vi "RGBC_readColour.vi"(8 "error in (no error)":errorcluster, 10 "channel":enum16{"clear", "red", "green", "blue"}(ring), 11 "I2C Ref In":T1={"myRIO Reference"={"myRIO Model"=enum."Unknown", "myRIO Hardware Reference"={"Generic FPGA Reference"=refnum, "Allow multiple opens"=FALSE}}, "I2C Channels Enum"=enum."Not Connected", "I2C Configuration"={"I2C Transfer Rate"=enum."Fast mode (400 kbps)"}}) -> (0 "error out":errorcluster, 1 "value":u8, 2 "Bytes Read":u8[](array[numeric]), 3 "I2C Ref Out":T1={"myRIO Reference"={"myRIO Model"=enum."Unknown", "myRIO Hardware Reference"={"Generic FPGA Reference"=refnum, "Allow multiple opens"=FALSE}}, "I2C Channels Enum"=enum."Not Connected", "I2C Configuration"={"I2C Transfer Rate"=enum."Fast mode (400 kbps)"}})   [LabVIEW 2017]
uses:
  <vilib>/myRIO/Instrument Drivers/Onboard IO/I2C/typedefs/I2C Reference.ctl
  <vilib>/myRIO/Common/Instrument Driver Framework/Utilities/typedefs/myRIO Generic Hardware Reference.ctl
  <vilib>/myRIO/Common/Instrument Driver Framework/Utilities/typedefs/Hardware Version Enum.ctl
  <vilib>/myRIO/Common/Instrument Driver Framework/Utilities/typedefs/myRIO v1.0 Reference.ctl
  <vilib>/myRIO/Common/Instrument Driver Framework/Utilities/typedefs/Generic FPGA Reference.ctl
  <vilib>/myRIO/Common/Instrument Driver Framework/myRIO v1.0/I2C/typedefs/I2C Channels Enum.ctl
  <vilib>/myRIO/Instrument Drivers/Onboard IO/I2C/typedefs/I2C Configuration.ctl
  <vilib>/myRIO/Instrument Drivers/Onboard IO/I2C/typedefs/I2C Transfer Rate.ctl
  <vilib>/Utility/error.llb/Error Cluster From Error Code.vi
  <vilib>/myRIO/Common/Instrument Driver Framework/myRIO v1.0/I2C/vis/myRIO v1.0 Write I2C.vi
  <vilib>/myRIO/Common/Instrument Driver Framework/myRIO v1.0/I2C/vis/myRIO v1.0 Read I2C.vi
  <vilib>/myRIO/Instrument Drivers/Onboard IO/I2C/I2C.lvlib
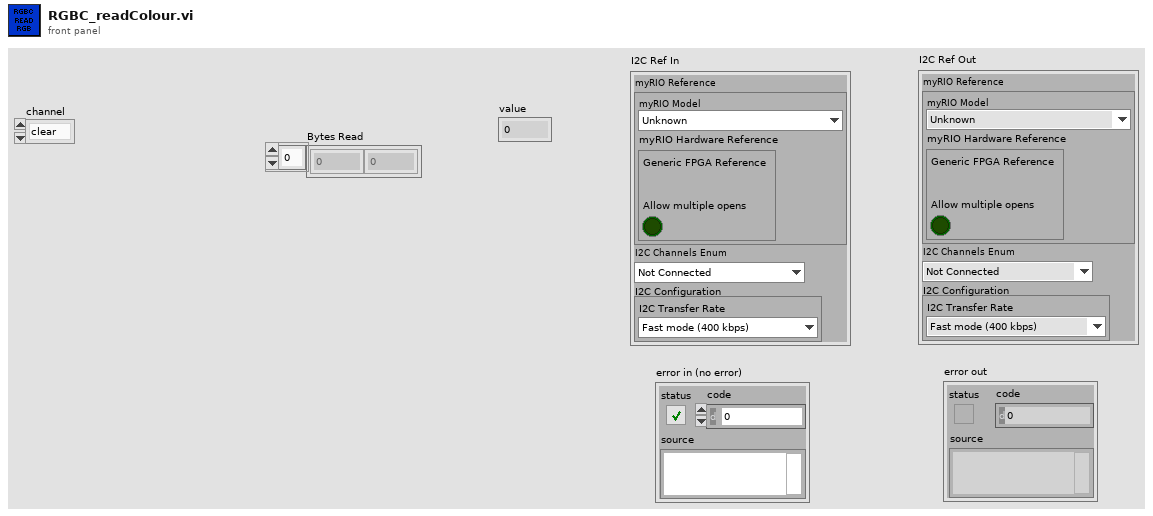
[diagram p1: front panel]
types:
  T1 = typedef "I2C.lvlib/I2C Reference.ctl" = cluster{"myRIO Reference":T2, "I2C Channels Enum":T6, "I2C Configuration":T7}
  T2 = typedef "myRIO Generic Hardware Reference.ctl" = cluster{"myRIO Model":T3, "myRIO Hardware Reference":T4}
  T3 = typedef "Hardware Version Enum.ctl" = enum16{"Unknown", "myRIO-1900", "myRIO-1950", "roboRIO", "NI ELVIS RIO CM"}
  T4 = typedef "myRIO v1.0 Reference.ctl" = cluster{"Generic FPGA Reference":T5, "Allow multiple opens":bool}
  T5 = typedef "Generic FPGA Reference.ctl" = refnum<k20>
  T6 = typedef "I2C Channels Enum.ctl" = enum16{"Not Connected", "A/I2C", "B/I2C", "I2C/I2C"}
  T7 = typedef "I2C.lvlib/I2C Configuration.ctl" = cluster{"I2C Transfer Rate":T8}
  T8 = typedef "I2C.lvlib/I2C Transfer Rate.ctl" = enum16{"Standard mode (100 kbps)", "Fast mode (400 kbps)"}
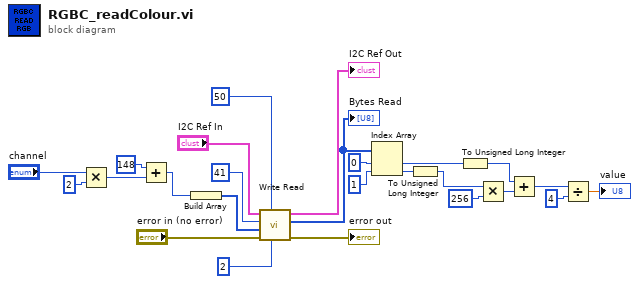
[diagram p0: block diagram]
diagram:
  n1 = Multiply(x="channel", y=2) -> (x*y=w17:i32)
  n2 = Add(x=u16 148, y=w17) -> (x+y=w14:i32)
  n3 = Build Array(w14) -> (w13:i32[])
  n4 = call <vilib>:"Write Read.vi"("Byte Count"=u32 2, "Timeout ms (1000)"=50, "error in (no error)"="error in (no error)", "Bytes to Write"=w13, "Slave Address (7-bit)"=u8 41, "I2C Ref In"="I2C Ref In") -> ("error out"=→"error out":errorcluster, "Bytes Read"=w12:u8[], "I2C Ref Out"=→"I2C Ref Out":T1)  [unwired: 2 in]
  "Bytes Read" <- w12
  n5 = Index Array(array=w12, index #1=0 ("index"), index #2=1 ("index")) -> (element #1=w9:u8, element #2=w8:u8)
  n6 = To Unsigned Long Integer(number=w8) -> (unsigned 32bit integer=w7:u32)
  n7 = To Unsigned Long Integer(number=w9) -> (unsigned 32bit integer=w4:u32)
  n8 = Multiply(x=w7, y=u32 256) -> (x*y=w5:u32)
  n9 = Add(x=w4, y=w5) -> (x+y=w3:u32)
  n10 = Divide(x=w3, y=u32 4) -> (x/y=→"value":dbl)
